vi "Shutdown.vi"(8 "error in (no error)":errorcluster, 11 "Config in":refnum<class "Config.lvclass">) -> (0 "error out":errorcluster, 3 "Config out":refnum<class "Config.lvclass">)   [LabVIEW 2019, in "Config.lvclass"]
doc: "Developed by Kevin Thompson\nkevin@thompsonengineering.net\n\nCopyright 2018-2020\nThompson Engineering, LLC"
uses:
  Config.lvclass
  Config.lvclass/Config.ctl
  Common/Startup/GBL System.vi
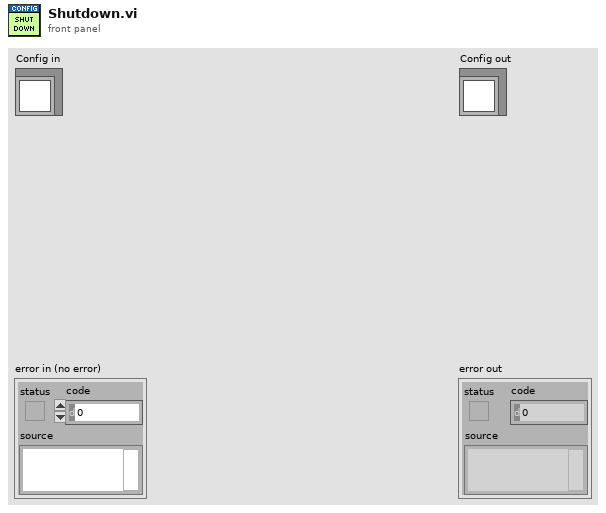
[diagram p1: front panel]
types:
  T1 = typedef "Config.lvclass/Config Settings.ctl" = cluster{"Application Settings":T2, "Main Settings":T3, "DAQ Settings":T6, "LogEngine Settings":T9}
  T2 = typedef "Application.lvclass/Settings--cluster.ctl" = cluster{"Simulation":bool}
  T3 = typedef "Main.lvclass/Settings--cluster.ctl" = cluster{"Simulation":bool, "Signal scaling":T4[], "ESR scaling":T5[], "num readings to average":i32[], "ESR alarm threshhold (%)":i32[], "UseDummyVrms":bool, "Dummy Vrms":dbl, "Inverter Database File":path, "default Inverter (name)":string[]}
  T4 = typedef "Main.lvclass/Gain control.ctl" = cluster{"Iin ripple gain":dbl, "Iout ripple gain":dbl, "Iout 60Hz gain ":dbl, "Vout 60Hz gain ":dbl, "Iin ripple offest":dbl, "Iout ripple offset":dbl, "Iout 60Hz offset":dbl, "Vout 60Hz offset":dbl}
  T5 = typedef "Main.lvclass/ESR scaling--cluster.ctl" = cluster{"Gain":dbl, "Offset":dbl}
  T6 = typedef "DAQ_Engine.lvclass/Settings--cluster.ctl" = cluster{"Simulation":bool, "Initial ErrReporting setting":i32, "Initial Measurement settings":T7, "Acquisition mode":T8, "DemoMode":bool, "RIO Device":string}
  T7 = typedef "Measurement Config--cluster.ctl" = cluster{"Data Rate 9775":dbl, "Data Rate 9215":dbl, "Samples RMS 9215":u32, "Samples RMS 9775":u32}
  T8 = typedef "Acquisition Mode--cluster.ctl" = enum16{"3phase", "Single"}
  T9 = typedef "Log_Engine.lvclass/Settings--cluster.ctl" = cluster{"Simulation":bool, "TDMS_FolderPath":string, "CSV_FolderPath":string, "TDMS_FileName_Prefix":string, "CSV_FileName_Prefix":string, "TDMS_LogDuration(s)":dbl, "CSV_LogDuration(s)":dbl}
  T10 = typedef "TD Pathnames--cluster.ctl" = cluster{"RunTimeSys?":bool, "AppFolder":path, "ExecutablePath":path, "ConfigFolder":path, "DataLogFolder":path, "SystemLogFolder":path, "SeqFolder":path, "MainStartupPathname":path, "MainUIPathname":path, "SystemEventsFile":path, "SeqEventsFile":path, "Config SettingsFile":path, "DAQ IOConfigFile":path, "SystemSimulation":bool}
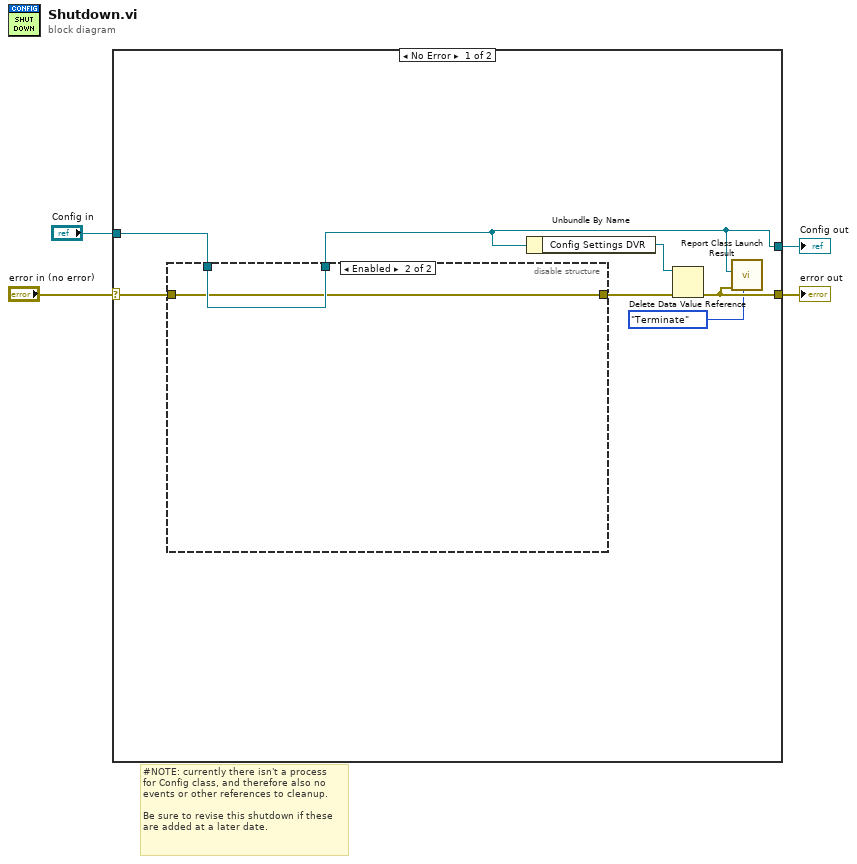
[diagram p0: block diagram]
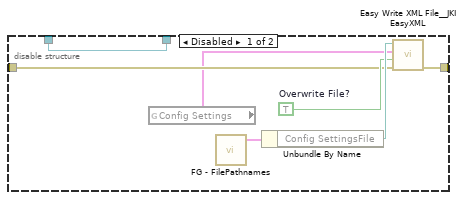
[diagram p2: hidden frame]
diagram:
  # "#NOTE: currently there isn't a process\nfor Config class, and therefore also no\nevents or other references to cleanup.\n\nBe sure to revise this shutdown if these\nare added at a later date."
  n1 = case shown="No Error" "error in (no error)" {
    selector: "error in (no error)" -> [w6 w22]
    tunnel: [w10 w22] -> w3
    tunnel: [w5 w21] -> w1
    tunnel: "Config in" -> [w8 w21]
    frame No Error {
      n2 = disable-structure shown="Enabled" {
        disable-tunnel: w8 -> [w14 w20]
        disable-tunnel: [w16 w19] -> w7
        disable-tunnel: w6 -> [w13 w19]
        disable-tunnel: [w14 w20] -> w5
        frame Disabled {
          w15 = TRUE  # Overwrite File?
          n3 = global read "GBL System.vi" "Config Settings"() -> (w12:T1)
          n4 = call "FG - FilePathnames.vi"() -> ("FilePaths out"=w18:T10)  [unwired: 4 in, 1 out]
          n5 = Unbundle By Name(w18) -> ("Config SettingsFile"=w17:path)
          n6 = call <vilib>:"Easy Write XML File__JKI EasyXML.vi"("error in (no error)"=w13, "Overwrite File? (false)"=w15, "LabVIEW Data"=w12, "XML File Path"=w17) -> ("error out"=w16:errorcluster)  [unwired: 6 in, 1 out]
        }
        frame Enabled {
        }
      }
      n7 = Unbundle By Name(w5) -> ("Config Settings DVR"=w11:refnum<data-value>)
      n8 = Delete Data Value Reference(data value reference=w11, error in=w7) -> (error out=w10:errorcluster)  [unwired: 1 out]
      n9 = call "Report Class Launch Result.vi"("Object"=w5, "error in (no error)"=w10, "Mode (Launch)"=enum16{"Launch", "Terminate"}."Terminate") -> ()  [unwired: 7 in, 1 out]
    }
    frame Error {
    }
  }
  "error out" <- w3
  "Config out" <- w1
